vi "_AdjustDataWithMode.vi"(9 "Action in":T1 caption="Action", 10 "Display State In in":T2 caption="State", 11 "Data In in":T5) -> (1 "Action out":T1 caption="Action", 2 "Display State In out":T2 caption="State", 3 "Data In out":T5)   [LabVIEW 2017, in "UI_TimeSelector.xctl"]
uses:
  UI_TimeSelector.xctl
  Data.ctl
  State.ctl
  Typedefs/INTERNAL-DATA.ctl
  Interface/DEF-Mode.ctl
  <vilib>/_xctls/Action.ctl
  <vilib>/_xctls/XControlSupport.lvlib
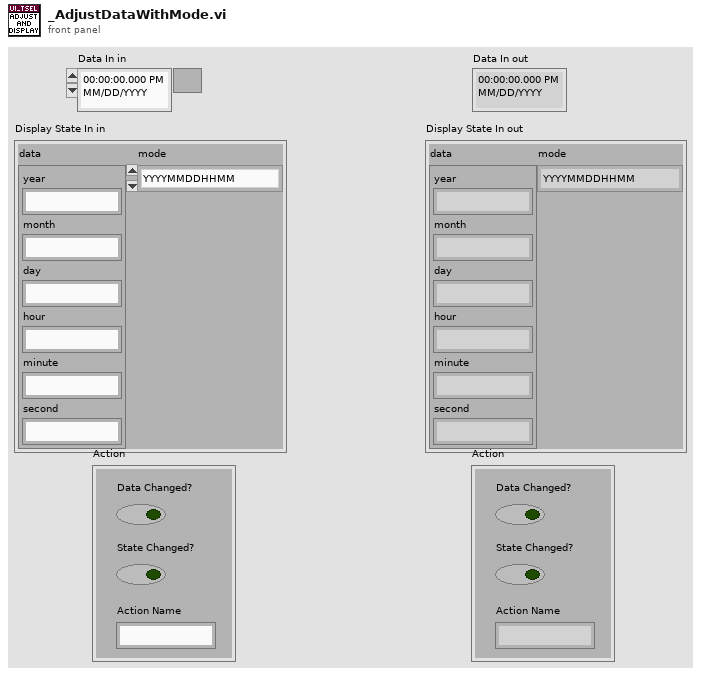
[diagram p1: front panel]
types:
  T1 = typedef "XControlSupport.lvlib/Action.ctl" = cluster{"Data Changed?":bool, "State Changed?":bool, "Action Name":string}
  T2 = typedef "UI_TimeSelector.xctl/State.ctl" = cluster{"data":T3, "mode":T4}
  T3 = typedef "UI_TimeSelector.xctl/INTERNAL-DATA.ctl" = cluster{"year":string, "month":string, "day":string, "hour":string, "minute":string, "second":string}
  T4 = typedef "UI_TimeSelector.xctl/DEF-Mode.ctl" = enum16{"YYYYMMDDHHMM", "YYYYMMDDHHMMSS", "YYYY", "YYYYMM", "YYYYMMDD", "HHMM", "HHMMSS"}
  T5 = typedef "UI_TimeSelector.xctl/Data.ctl" = timestamp
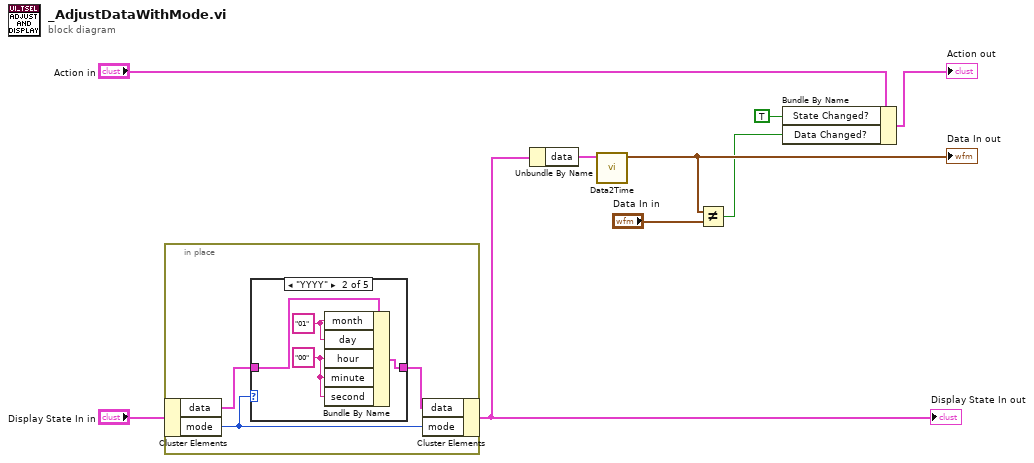
[diagram p0: block diagram]
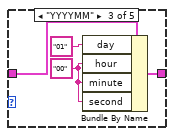
[diagram p3: hidden frame]
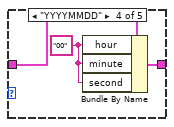
[diagram p4: hidden frame]
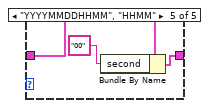
[diagram p5: hidden frame]
diagram:
  n1 = in-place {
    n2 = in-place-cluster #1("Display State In in") -> ("data"=w11:T3, "mode"=w12:T4)
    n3 = case shown="\"YYYY\"" w12 {
      tunnel: w11 -> [w13 w17 w19 w23 w27]
      tunnel: [w13 w16 w18 w22 w26] -> w10
      frame "YYYYMMDDHHMMSS", "HHMMSS", Default {
      }
      frame "YYYY" {
        w14 = "01" ("hour")
        w15 = "00" ("hour")
        n4 = Bundle By Name(cluster=w17, "month"=w14, "day"=w14, "hour"=w15, "minute"=w15, "second"=w15) -> (w16:T3)
      }
      frame "YYYYMM" {
        w21 = "00" ("hour")
        n5 = Bundle By Name(cluster=w19, "day"="01" ("hour"), "hour"=w21, "minute"=w21, "second"=w21) -> (w18:T3)
      }
      frame "YYYYMMDD" {
        w24 = "00" ("hour")
        n6 = Bundle By Name(cluster=w23, "hour"=w24, "minute"=w24, "second"=w24) -> (w22:T3)
      }
      frame "YYYYMMDDHHMM", "HHMM" {
        n7 = Bundle By Name(cluster=w27, "second"="00" ("hour")) -> (w26:T3)
      }
    }
    n8 = in-place-cluster #1("data"=w10, "mode"=w12) -> (w9:T2)
  }
  "Display State In out" <- w9
  n9 = Unbundle By Name(w9) -> ("data"=w5:T3)
  n10 = call "Data2Time.vi"("data"=w5) -> ("Time"=w3:timestamp)  [unwired: 10 in]
  "Data In out" <- w3
  n11 = Not Equal?(x=w3, y="Data In in") -> (x != y?=w2:bool)
  n12 = Bundle By Name(cluster="Action in", "State Changed?"=TRUE, "Data Changed?"=w2) -> (→"Action out":T1)
